vi "readFromXMLFile.vi"() -> ()   [LabVIEW 2017]
panel:
  in  "count":i32
  out "appended array":string[](array[string])
  out "cancelled":bool
  in  "file (use dialog)":path
  in  "error in":errorcluster
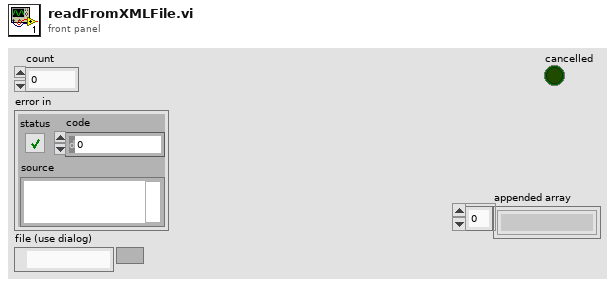
[diagram p1: front panel]
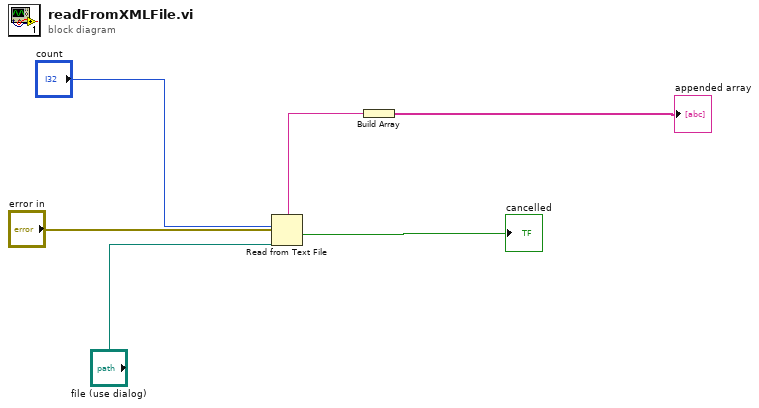
[diagram p0: block diagram]
diagram:
  n1 = Read from Text File(file (use dialog)="file (use dialog)", count="count", error in="error in") -> (text=w3:string, cancelled=→"cancelled":bool)  [unwired: 1 in, 2 out]
  n2 = Build Array(w3) -> (→"appended array":string[])
